vi "JSON Config Unit Tests.vi"(8 "error in (no error)":errorcluster) -> (0 "error out":errorcluster)   [LabVIEW 2021]
uses:
  Source/Abs_Types/Double Float/Abs_Double Float.lvclass
  C:/New folder/LV_Abstract/LV_Abstract/Source/Abs_Types/Type/Abs_Type.lvclass
  Source/Abs_Types/Extended Float/Abs_Extended Float.lvclass
  Source/Abs_Types/Single Float/Abs_Single Float.lvclass
  Source/Abs_Types/Time/Abs_Time.lvclass
  Source/Abs_Types/I8 Integer/Abs_I8 Integer.lvclass
  Source/Abs_Types/I16 Integer/Abs_I16 Integer.lvclass
  Source/Abs_Types/I32 Integer/Abs_I32 Integer.lvclass
  Source/Abs_Types/I64 Integer/Abs_I64 Integer.lvclass
  Source/Abs_Types/U8 Integer/Abs_U8 Integer.lvclass
  Source/Abs_Types/U16 Integer/Abs_U16 Integer.lvclass
  Source/Abs_Types/U32 Integer/Abs_U32 Integer.lvclass
  Source/Abs_Types/U64 Integer/Abs_U64 Integer.lvclass
  Source/Abs_Types/Boolean/Abs_Boolean.lvclass
  Source/Abs_Types/String/Abs_String.lvclass
  <vilib>/numeric/Random Number (Range) DBL.vi
  f7d354b6-3130-4a28-b63b-0f072b3279d1.vi
  0ce517fe-5015-4783-ac61-4d8fd32a6602.vi
  5b325d72-b577-47c1-812e-23417f3b633e.vi
  5617c745-7de0-4ce6-b875-a3b8f4132d17.vi
  9756081b-5807-4c67-a150-855992f423cf.vi
  6efb0f4b-b48c-495c-b974-5a8ae3dddfee.vi
  6ffe79a1-e932-4601-93c7-2041e8fb7702.vi
  4c3d59d5-1451-4628-b6b2-b86360b8c9b4.vi
  3a7515f3-65d7-4d64-bff9-d0c5544e8f28.vi
  ce9be0dc-0286-421a-9039-997fd818a233.vi
  da359710-7a58-4dc9-aef9-415f89e65867.vi
  Source/Abs_Types/Abs_Simple_Read.vi
  Source/Abs_Types/Boolean/Simple Read.vi
  Source/Abs_Types/String/Simple Read.vi
  Source/Abs_Types/Double Float/Simple Read.vi
  Source/Abs_Types/Extended Float/Simple Read.vi
  Source/Abs_Types/Single Float/Simple Read.vi
  Source/Abs_Types/I8 Integer/Simple Read.vi
  Source/Abs_Types/I16 Integer/Simple Read.vi
  Source/Abs_Types/I32 Integer/Simple Read.vi
  Source/Abs_Types/I64 Integer/Simple Read.vi
  Source/Abs_Types/U8 Integer/Simple Read.vi
  Source/Abs_Types/U16 Integer/Simple Read.vi
  Source/Abs_Types/U32 Integer/Simple Read.vi
  Source/Abs_Types/U64 Integer/Simple Read.vi
  <vilib>/Utility/Data Type/Get Type Information.vi
  Source/Constants/Abs_Constant.vi
  Source/Constants/Support/Bool/Bool.vi
  <vilib>/addons/_JKI Toolkits/Caraya/classes/Test/Define Test.vi
  Source/Abs_Types/Type/Read Config JSON.vi
  <vilib>/addons/_JKI Toolkits/Caraya/classes/Assert/Assert.vi
  <vilib>/addons/_JKI Toolkits/Caraya/classes/Assert/Assert Equal Value_Variant.vi
  <vilib>/addons/_JKI Toolkits/Caraya/classes/Assert/Assert Equal Type_Variant.vi
  Source/Constants/Support/Str/Str.vi
  Source/Constants/Support/DBL/DBL.vi
  <vilib>/addons/_JKI Toolkits/Caraya/classes/Assert/Assert Almost Equal_Float.vi
  Source/Constants/Support/EXT/EXT.vi
  Source/Constants/Support/SGL/SGL.vi
  Source/Constants/Support/I8/I8.vi
  Source/Constants/Support/I16/I16.vi
  Source/Constants/Support/I32/I32.vi
  Source/Constants/Support/I64/I64.vi
  Source/Constants/Support/U8/U8.vi
  Source/Constants/Support/U16/U16.vi
  Source/Constants/Support/U32/U32.vi
  Source/Constants/Support/U64/U64.vi
  Source/Constants/Support/DBL/Const_DBL.lvclass
  Source/Constants/Support/U8/Const_U8.lvclass
  Source/Constants/Support/U16/Const_U16.lvclass
  Source/Constants/Support/U32/Const_U32.lvclass
  Source/Constants/Support/U64/Const_U64.lvclass
  Source/Abs_Types/Complex Double Float/Abs_Complex Double Float.lvclass
  Source/Abs_Types/Complex Extended Float/Abs_Complex Extended Float.lvclass
  Source/Abs_Types/Complex Single Float/Abs_Complex Single Float.lvclass
  39f596e4-2794-4729-acf7-f3e07dc76b0e.vi
  91ca4360-0577-4b01-ad6f-e6f8a251b182.vi
  18f5e6da-b008-4c23-b7d3-f76676ecceac.vi
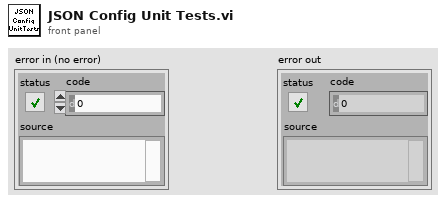
[diagram p1: front panel]
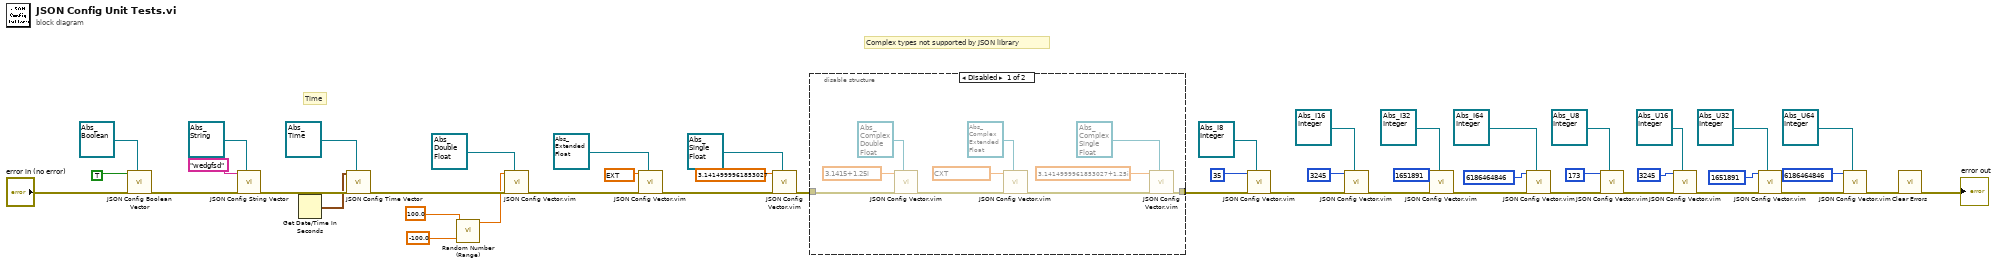
[diagram p0: block diagram]
diagram:
  # "Complex types not supported by JSON library"
  # "Time"
  n1 = call "JSON Config Boolean Vector.vi"("Class"=refnum<class "Abs_Boolean.lvclass"> refnum ("Abs_Boolean.lvclass"), "error in (no error)"="error in (no error)", "Test Value"=TRUE) -> ("error out"=w1:errorcluster)  [unwired: 8 in]
  n2 = call "JSON Config String Vector.vi"("Class"=refnum<class "Abs_String.lvclass"> refnum ("Abs_String.lvclass"), "error in (no error)"=w1, "Test Value"="wedgfsd") -> ("error out"=w40:errorcluster)  [unwired: 8 in]
  n3 = Get Date/Time In Seconds() -> (seconds since 1Jan1904=w37:timestamp)
  n4 = call "JSON Config Time Vector.vi"("Expected Class"=refnum<class "Abs_Time.lvclass"> refnum ("Abs_Time.lvclass"), "error in (no error)"=w40, "Test Value"=w37) -> ("error out"=w39:errorcluster)  [unwired: 8 in]
  n5 = call-poly <vilib>:"Random Number (Range).vi"("lower bound (0)"=-100.0, "upper bound (100)"=100.0) -> ("number"=w8:dbl)  [unwired: 9 in]
  n6 = call "JSON Config Vector.vim"("Class"=refnum<class "Abs_Double Float.lvclass"> refnum, "error in (no error)"=w39, "Test Value"=w8) -> ("error out"=w46:errorcluster)  [unwired: 8 in]
  n7 = call "JSON Config Vector.vim"("Class"=refnum<class "Abs_Extended Float.lvclass"> refnum ("Abs_Extended Float.lvclass"), "error in (no error)"=w46, "Test Value"=ext 3.1414999999999999999) -> ("error out"=w42:errorcluster)  [unwired: 8 in]
  n8 = call "JSON Config Vector.vim"("Class"=refnum<class "Abs_Single Float.lvclass"> refnum ("Abs_Single Float.lvclass"), "error in (no error)"=w42, "Test Value"=sgl 3.1415) -> ("error out"=w36:errorcluster)  [unwired: 8 in]
  n9 = disable-structure shown="Disabled" {
    disable-tunnel: w36 -> [w56 w58]
    disable-tunnel: [w48 w58] -> w35
    frame Disabled {
      n10 = call "JSON Config Vector.vim"("Class"=refnum<class "Abs_Complex Double Float.lvclass"> refnum ("Abs_Complex Double Float.lvclass"), "error in (no error)"=w56, "Test Value"=cdb 3.1415+1.25i) -> ("error out"=w53:errorcluster)  [unwired: 8 in]
      n11 = call "JSON Config Vector.vim"("Class"=refnum<class "Abs_Complex Extended Float.lvclass"> refnum ("Abs_Complex Extended Float.lvclass"), "error in (no error)"=w53, "Test Value"=cxt 3.1415+1.25i) -> ("error out"=w50:errorcluster)  [unwired: 8 in]
      n12 = call "JSON Config Vector.vim"("Class"=refnum<class "Abs_Complex Single Float.lvclass"> refnum ("Abs_Complex Single Float.lvclass"), "error in (no error)"=w50, "Test Value"=csg 3.1415+1.25i) -> ("error out"=w48:errorcluster)  [unwired: 8 in]
    }
    frame Enabled {
    }
  }
  n13 = call "JSON Config Vector.vim"("Class"=refnum<class "Abs_I8 Integer.lvclass"> refnum ("Abs_I8 Integer.lvclass"), "error in (no error)"=w35, "Test Value"=i8 35) -> ("error out"=w31:errorcluster)  [unwired: 8 in]
  n14 = call "JSON Config Vector.vim"("Class"=refnum<class "Abs_I16 Integer.lvclass"> refnum ("Abs_I16 Integer.lvclass"), "error in (no error)"=w31, "Test Value"=i16 3245) -> ("error out"=w28:errorcluster)  [unwired: 8 in]
  n15 = call "JSON Config Vector.vim"("Class"=refnum<class "Abs_I32 Integer.lvclass"> refnum ("Abs_I32 Integer.lvclass"), "error in (no error)"=w28, "Test Value"=1651891) -> ("error out"=w25:errorcluster)  [unwired: 8 in]
  n16 = call "JSON Config Vector.vim"("Class"=refnum<class "Abs_I64 Integer.lvclass"> refnum ("Abs_I64 Integer.lvclass"), "error in (no error)"=w25, "Test Value"=i64 6186464846) -> ("error out"=w22:errorcluster)  [unwired: 8 in]
  n17 = call "JSON Config Vector.vim"("Class"=refnum<class "Abs_U8 Integer.lvclass"> refnum ("Abs_U8 Integer.lvclass"), "error in (no error)"=w22, "Test Value"=u8 173) -> ("error out"=w20:errorcluster)  [unwired: 8 in]
  n18 = call "JSON Config Vector.vim"("Class"=refnum<class "Abs_U16 Integer.lvclass"> refnum ("Abs_U16 Integer.lvclass"), "error in (no error)"=w20, "Test Value"=u16 3245) -> ("error out"=w17:errorcluster)  [unwired: 8 in]
  n19 = call "JSON Config Vector.vim"("Class"=refnum<class "Abs_U32 Integer.lvclass"> refnum ("Abs_U32 Integer.lvclass"), "error in (no error)"=w17, "Test Value"=u32 1651891) -> ("error out"=w14:errorcluster)  [unwired: 8 in]
  n20 = call "JSON Config Vector.vim"("Class"=refnum<class "Abs_U64 Integer.lvclass"> refnum ("Abs_U64 Integer.lvclass"), "error in (no error)"=w14, "Test Value"=u64 6186464846) -> ("error out"=w11:errorcluster)  [unwired: 8 in]
  n21 = call <vilib>:"Clear Errors.vi"("error in (no error)"=w11) -> ("error out"=→"error out":errorcluster)  [unwired: 5 in, 1 out]
